vi "Decoder.vi"(0 "Реле in":bool, 1 "Реле 3":bool, 2 "Реле 4":bool, 3 "Токоограничитель":bool, 5 "Повторы(0..255)":u8=1, 7 "Начальное напряжение(0..255)":u8, 9 "Задержка (10 мс)(0..255)":u8=1, 11 "50 герцовый фильтр":bool, 12 "Реле 1":bool, 13 "Диапазон напряжения(0..255)":u8=255, 14 "Количество шагов(0..255)":u8=255) -> (4 "string":string)   [LabVIEW 2013]
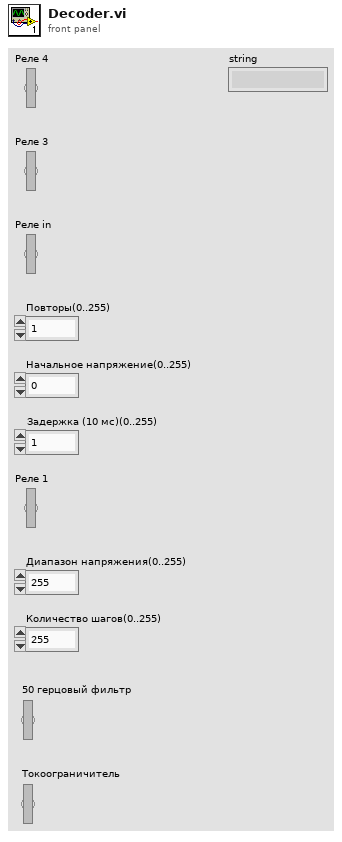
[diagram p1: front panel]
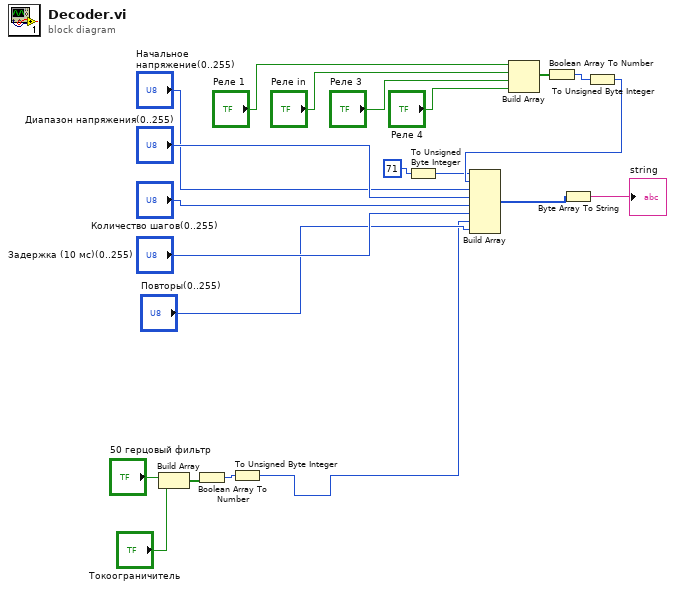
[diagram p0: block diagram]
diagram:
  n1 = Build Array("50 герцовый фильтр", "Токоограничитель") -> (w5:bool[])
  n2 = Boolean Array To Number(Boolean array=w5) -> (number=w4:u32)
  n3 = To Unsigned Byte Integer(number=w4) -> (unsigned 8bit integer=w1:u8)
  n4 = To Unsigned Byte Integer(number=71) -> (unsigned 8bit integer=w19:u8)
  n5 = Build Array("Реле 1", "Реле in", "Реле 3", "Реле 4") -> (w15:bool[])
  n6 = Boolean Array To Number(Boolean array=w15) -> (number=w20:u32)
  n7 = To Unsigned Byte Integer(number=w20) -> (unsigned 8bit integer=w21:u8)
  n8 = Build Array(w19, w21, "Начальное напряжение(0..255)", "Диапазон напряжения(0..255)", "Количество шагов(0..255)", "Задержка (10 мс)(0..255)", w1, "Повторы(0..255)") -> (w16:u8[])
  n9 = Byte Array To String(unsigned byte array=w16) -> (string=→"string":string)
